vi "Delete User.vi"(8 "error in":errorcluster, 10 "Multicolumn Listbox":i32(listbox), 11 "Path":path=path "C:/Users/subasrees/Desktop/New folder/abcd.xls") -> (0 "error out":errorcluster)   [LabVIEW 2015]
uses:
  <vilib>/Utility/file.llb/Read Delimited Spreadsheet (string).vi
  <vilib>/Utility/file.llb/Write Delimited Spreadsheet (string).vi
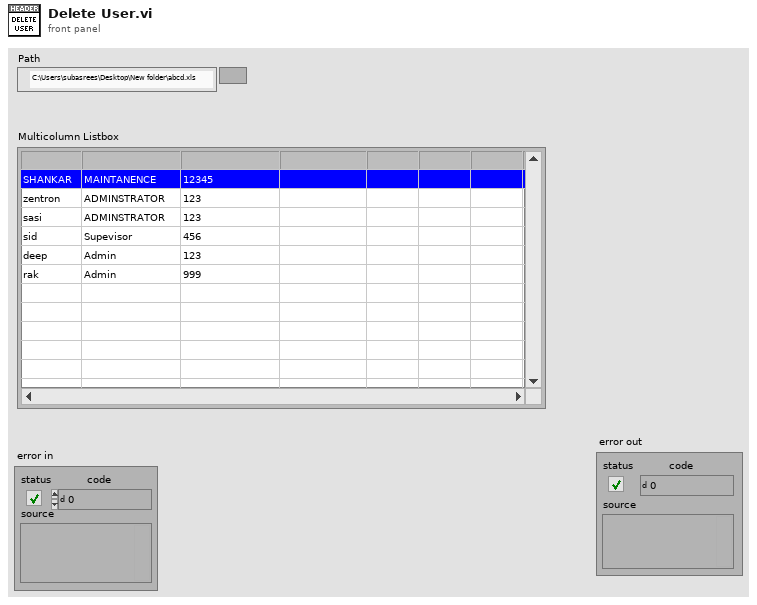
[diagram p1: front panel]
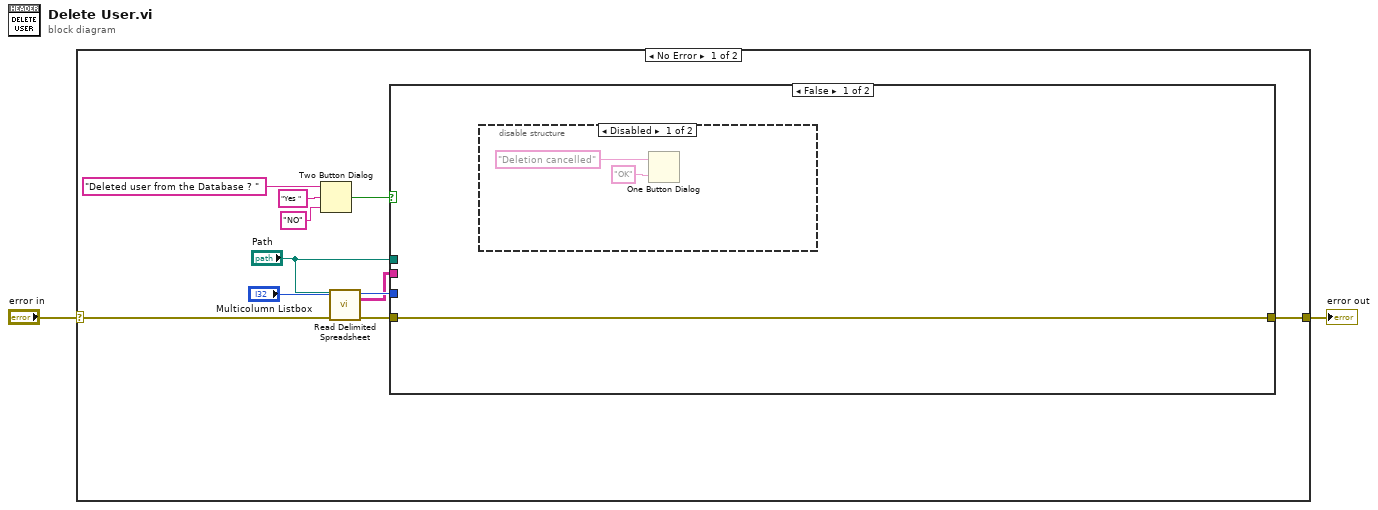
[diagram p0: block diagram]
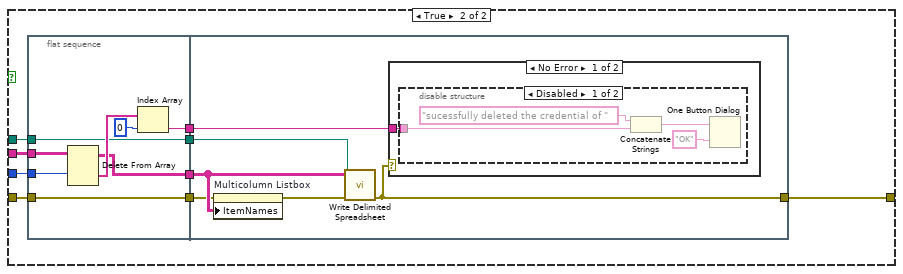
[diagram p3: hidden frame]
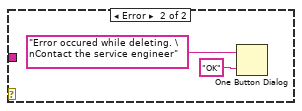
[diagram p5: hidden frame]
diagram:
  n1 = case shown="No Error" "error in" {
    selector: "error in" -> [w4 w46]
    tunnel: [w3 w46] -> w1
    frame No Error {
      n2 = Two Button Dialog(message="Deleted user from the Database ? ", 1:"NO" ("F button name (\"Cancel\")"), 2:"Yes " ("T button name (\"OK\")")) -> (T button?=w8:bool)
      n3 = call-poly <vilib>:"Read Delimited Spreadsheet.vi"("file path (dialog if empty)"="Path", "error in (no error)"=w4) -> ("all rows"=w6:string[][], "error out"=w5:errorcluster)  [unwired: 8 in, 4 out]
      n4 = case shown="False" w8 {
        tunnel: w6 -> [_ w21]
        tunnel: "Path" -> [_ w20]
        tunnel: "Multicolumn Listbox" -> [_ w19]
        tunnel: [w13 w18] -> w3
        tunnel: w5 -> [w13 w17]
        frame False {
          n5 = disable-structure shown="Disabled" {
            frame Disabled {
              n6 = One Button Dialog(message="Deletion cancelled", button name ("OK")="OK") -> ()  [unwired: 1 out]
            }
            frame Enabled {
            }
          }
        }
        frame True {
          n7 = flat-sequence {
            tunnel: [w28] -> w24
            tunnel: [w29] -> w23
            tunnel: [w30] -> w22
            tunnel: w21 -> [w26]
            tunnel: w20 -> [w28]
            tunnel: w19 -> [w27]
            tunnel: w17 -> [w25]
            tunnel: [w25] -> w16
            tunnel: w24 -> [w33]
            tunnel: w23 -> [w37]
            tunnel: w22 -> [w38]
            tunnel: [w34] -> w18
            tunnel: w16 -> [w36]
            frame #0 {
              n8 = Delete From Array(array=w26, index (row)=w27) -> (deleted portion=w32:string[], array with subset deleted=w29:string[][])  [unwired: 2 in]
              n9 = Index Array(array=w32, index=0) -> (element=w30:string)
            }
            frame #1 {
              n10 = property on="Multicolumn Listbox" class="MCListbox (strict)"(error in=w36, "ItemNames"=w37) -> (error out=w35:errorcluster)  [unwired: 1 in, 1 out]
              n11 = call-poly <vilib>:"Write Delimited Spreadsheet.vi"("file path (dialog if empty)"=w33, "2D data"=w37, "error in (no error)"=w35) -> ("error out"=w34:errorcluster)  [unwired: 11 in, 1 out]
              n12 = case shown="No Error" w34 {
                tunnel: w38 -> [w39 _]
                frame No Error {
                  n13 = disable-structure shown="Disabled" {
                    disable-tunnel: w39 -> [w42 _]
                    frame Disabled {
                      n14 = Concatenate Strings("sucessfully deleted the credential of " ("message"), w42) -> (w41:string)
                      n15 = One Button Dialog(message=w41, button name ("OK")="OK") -> ()  [unwired: 1 out]
                    }
                    frame Enabled {
                    }
                  }
                }
                frame Error {
                  n16 = One Button Dialog(message="Error occured while deleting. \nContact the service engineer", button name ("OK")="OK") -> ()  [unwired: 1 out]
                }
              }
            }
          }
        }
      }
    }
    frame Error {
    }
  }
  "error out" <- w1
